vi "Read Network Protocol.vi"(8 "error in (no error)":errorcluster, 11 "Master CR in":refnum<class "Master CR.lvclass">) -> (0 "error out":errorcluster, 2 "Network Protocol":refnum<class "Network Protocol.lvclass">, 3 "Master CR out":refnum<class "Master CR.lvclass">)   [LabVIEW 2021, in "Master CR.lvclass"]
uses:
  Master CR.lvclass
  Modbus_v121c/Network Protocol/Network Protocol.lvclass
  Master CR.lvclass/Master CR.ctl
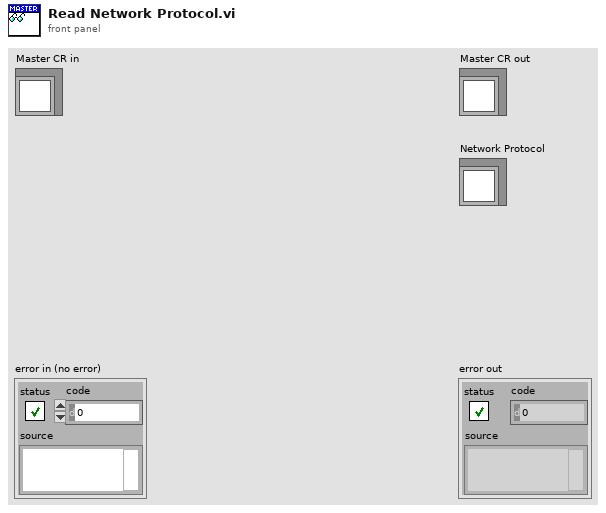
[diagram p1: front panel]
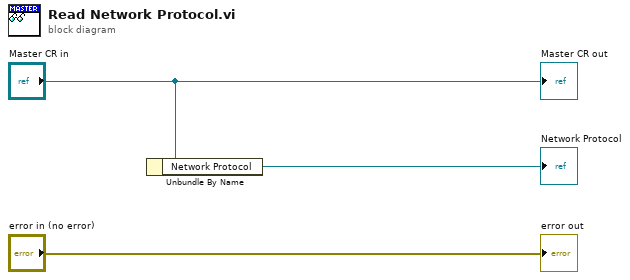
[diagram p0: block diagram]
diagram:
  n1 = Unbundle By Name("Master CR in") -> ("Network Protocol"=→"Network Protocol":refnum<class "Network Protocol.lvclass">)
  "error out" <- "error in (no error)"
  "Master CR out" <- "Master CR in"
